vi "Save to ActiveX Excel - v2b.vi"(0 "Path":path caption="Excel Path", 1 "Excel._SheetName":string, 2 "ErrorIn":errorcluster, 3 "Ikol":i32, 4 "Table Mean Data":dbl[][](array[numeric])=[[0.03982848859388113, 0.8783843747615788, 1.7307777523460754, 2.548700999465932, 3.364561226825355], [0.09683070115205593, 0.9242182040131244, 1.7732014953841466, 2.5928838025482537, 3.4105195696955795], [0.13037125200274627, 0.9741591515983836, 1.8122639810788133, 2.646598611429008, 3.4407147325856373], [0.3228925001907382, 1.1797897306782663, 2.005814297703518, 2.8300938429846627, 3.6218649576562103], [0.3520146486610215, 1.202849774929428, 2.0447998779278245, 2.863716182192717, 3.6558284885938757], [1.3171953917753891, 2.1611230640115955, 2.9585827420462296, 3.7653595788509917, 4.528567025253687], [1.462092622262916, 2.2864551766231758, 3.104032959487296, 3.888673838406958, 4.6586440833142655], [1.5022079804684525, 2.335135728999771, 3.1296809338521387, 3.9336214236667435, 4.6988430609598], [1.5266187533379127, 2.364577096208133, 3.181790493629352, 3.9747548638132284, 4.713216449225604], [1.579623102159153, 2.4058289463645393, 3.208687266346226, 3.998727397573815, 4.759391470206768], [1.5989642175936543, 2.438834210727091, 3.2499842832074437, 4.027358205539025, 4.791335317006178], [1.6367565423056383, 2.4624704356450744, 3.273314106965741, 4.061460288395512, 4.821456626230265], [1.671589227130543, 2.5053598840314315, 3.307654840924691, 4.078201876859696, 4.83912291142138], [1.9548839551384747, 2.773676356145566, 3.5854721904325912, 4.353372701609829, 5.09703150988022], [1.9735957885099578, 2.8088496223392054, 3.6178268101014686, 4.38579995422294, 5.1040573739223385], [2.0215237659266037, 2.8251621271076495, 3.645978484779123, 4.413374227512019, 5.154262607766843], [2.063611200122071, 2.874846112764169, 3.6707408255130813, 4.4413080033569905, 5.182666971847107], [2.079061264972915, 2.9107945372701596, 3.7083878843366103, 4.474929121843292, 5.207357900358588], [2.3204461738002595, 3.1260236514839432, 3.9160466926070003, 4.67015243762875, 5.400686655985356], [2.4909175249866458, 3.2829407186999267, 4.078123140306708, 4.827607843137255, 5.545498435950253], [2.5371688410772846, 3.333136186770425, 4.0956087586785666, 4.86724528877699, 5.5768307011520575], [2.5549810025177377, 3.3498875410086164, 4.146593423361565, 4.901781948577098, 5.606005340657667], [2.593616845960172, 3.384173342488744, 4.175310292210271, 4.926442969405671, 5.625553368429085], [2.619952697032122, 3.4272117189288145, 4.190040131227593, 4.949809414816512, 5.647464713511864], [2.653675135423816, 3.450658121614398, 4.245682459754332, 4.983065537499049, 5.691289234760052], [2.856990615701531, 3.658316319523915, 4.410946211947819, 5.168084229800873, 5.859205615320062], [2.8970571450369995, 3.693769130998695, 4.459168383306632, 5.196810254062712, 5.892754711223012], [2.9354152742809165, 3.724582589456009, 4.481760280766007, 5.235593804837112, 5.9293153276874975], [4.518166475928902, 5.240471808957046, 5.927615472648206, 6.580137026016633, 7.176726939803161], [4.664593881132227, 5.399151598382549, 6.073597314412142, 6.700255436026549, 7.293027542534518], [4.6941597619592645, 5.413944914930952, 6.0971688410772895, 6.732541084916453, 7.310430151827263], [4.72799206530862, 5.443506523231869, 6.131480888075072, 6.7552147707331915, 7.341015335316998], [4.7442490272373625, 5.474857709620816, 6.148384832532239, 6.7895329213397355, 7.36304692149233], [4.777299458304725, 5.499158617532617, 6.170540321965362, 6.816587167162586, 7.378775310902568], [4.798946517128253, 5.526323338673995, 6.192271610589764, 6.82118928816662, 7.387563897154188], [4.901620202944993, 5.615843137254902, 6.292097352559698, 6.903707026779581, 7.473250629434656], [4.92828442816816, 5.6507722590981935, 6.304925917448693, 6.934254978255892, 7.480664072632936], [4.969151140611893, 5.675261158159765, 6.339691462577246, 6.9630627908751, 7.530664835584031], [5.006560158693834, 5.692798657206076, 6.368715953307389, 6.9916246280613334, 7.535613031204692], [5.044118715190357, 5.727861448081179, 6.395839169909206, 7.010927901121539, 7.563150072480349], [5.057027237354088, 5.78310582131685, 6.423008773937592, 7.0214792095826635, 7.583959105821311], [5.089166399633788, 5.78664469367514, 6.443226367589837, 7.063651483939874, 7.6117824063477455], [5.118777447165641, 5.826187533379106, 6.48167971313039, 7.071441519798577, 7.6265043106736785], [5.147915465018696, 5.842330357824063, 6.504778820477606, 7.0906581216144, 7.640489509422445], [5.195048142214084, 5.883804379339284, 6.519934691386284, 7.136523079270609, 7.677748378728906], [5.348665598535132, 6.047138780804155, 6.676741893644613, 7.253650110627901, 7.78973495078965], [5.394423743038073, 6.086649881742575, 6.72477546349278, 7.303063096055544, 7.841829861905848], [5.41259601739528, 6.1073417257953695, 6.748100404364077, 7.307313649195082, 7.860812085145335]]) -> (5 "error out":errorcluster, 6 "OK":bool)   [LabVIEW 2018]
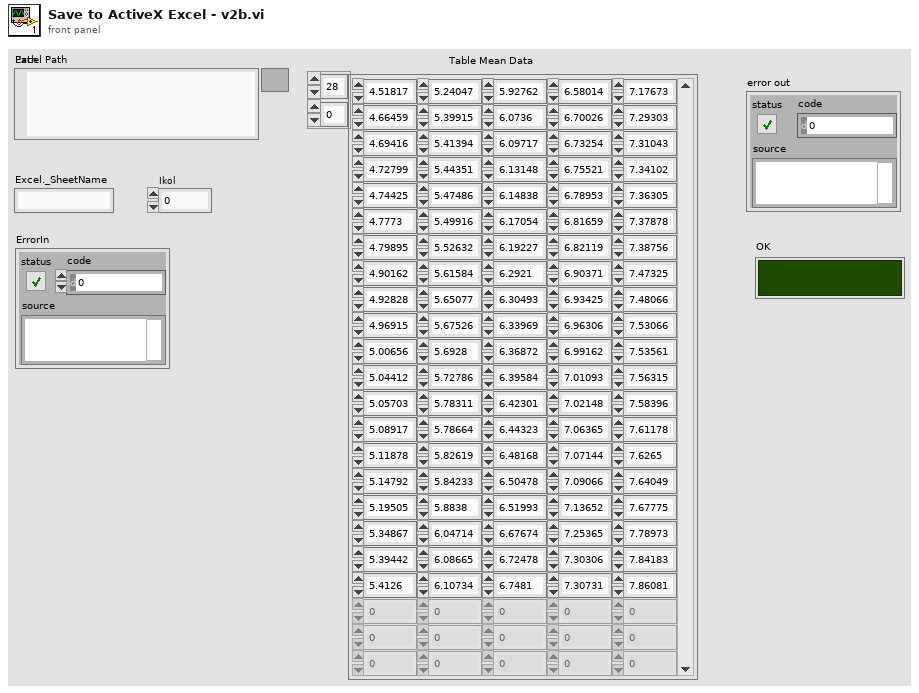
[diagram p1: front panel]
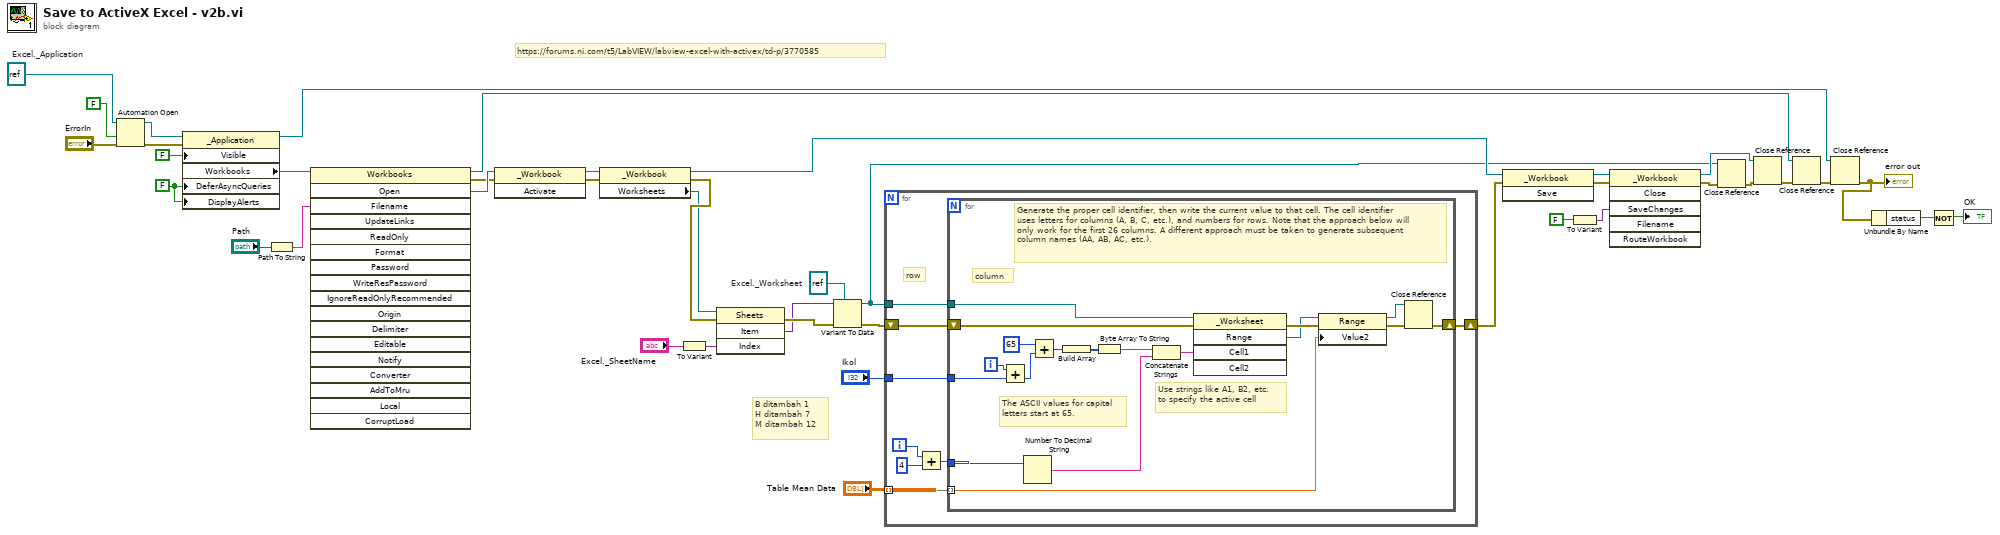
[diagram p0: block diagram]
diagram:
  w10 = refnum<k7> refnum  # Excel._Worksheet
  w41 = FALSE ("DeferAsyncQueries")
  w37 = refnum<k7> refnum  # Excel._Application
  # "B ditambah 1\nH ditambah 7\nM ditambah 12"
  # "https://forums.ni.com/t5/LabVIEW/labview-excel-with-activex/td-p/3770585"
  n1 = Automation Open(error in (no error)="ErrorIn", Automation Refnum=w37, 9:FALSE ("open new instance (false)")) -> (Automation Refnum=w39:refnum<k7>, error out=w38:errorcluster)  [unwired: 1 out]
  n2 = property class="_Application"(reference=w39, error in=w38, "Visible"=FALSE, "DeferAsyncQueries"=w41, "DisplayAlerts"=w41) -> (reference out=w17:refnum<k7>, "Workbooks"=w33:refnum<k7>)  [unwired: 1 out]
  n3 = Path To String(path="Path") -> (string=w30:string)
  n4 = invoke class="Workbooks" method="Open"(reference=w33, "Filename"=w30) -> (reference out=w19:refnum<k7>, error out=w34:errorcluster, "Open"=w35:refnum<k7>)  [unwired: 16 in, 15 out]
  n5 = invoke class="_Workbook" method="Activate"(reference=w35, error in=w34) -> (reference out=w29:refnum<k7>, error out=w28:errorcluster)  [unwired: 1 in, 1 out]
  n6 = property class="_Workbook"(reference=w29, error in=w28) -> (reference out=w27:refnum<k7>, error out=w4:errorcluster, "Worksheets"=w3:refnum<k7>)
  n7 = To Variant(anything="Excel._SheetName") -> (Variant=w6:variant)
  n8 = invoke class="Sheets" method="Item"(reference=w3, error in=w4, "Index"=w6) -> (error out=w5:errorcluster, "Item"=w2:variant)  [unwired: 1 in, 2 out]
  n9 = Variant To Data(error in=w5, type=w10, Variant=w2) -> (data=w8:refnum<k7>, error out=w12:errorcluster)
  n10 = for {
    shift-right: [w48] -> w9
    shift-left: w12 -> [w49]
    tunnel: w8 -> [w47]
    tunnel: "Table Mean Data" -> [w45] mode=indexing
    tunnel: "Ikol" -> [w42]
    i -> [w44]
    # "row"
    n11 = Add(x=w44, y=4) -> (x+y=w46:i32)
    n12 = for {
      shift-right: [w64] -> w48
      shift-left: w49 -> [w62]
      tunnel: w47 -> [w61]
      tunnel: w46 -> [w57]
      tunnel: w45 -> [w53] mode=indexing
      tunnel: w42 -> [w50]
      i -> [w51]
      # "column"
      # "Use strings like A1, B2, etc. to specify the active cell"
      # "The ASCII values for capital letters start at 65."
      # "Generate the proper cell identifier, then write the current value to that cell. The cell identifier uses letters for columns (A, B, C, etc.), and numbers for rows. Note that the approach below will only work for the first 26 columns. A different approach must be taken to generate subsequent column names (AA, AB, AC, etc.)."
      n13 = Add(x=w51, y=w50) -> (x+y=w52:i32)
      n14 = Number To Decimal String(number=w57) -> (decimal integer string=w55:string)  [unwired: 1 in]
      n15 = Add(x=65, y=w52) -> (x+y=w59:i32)
      n16 = Build Array(w59) -> (w58:i32[])
      n17 = Byte Array To String(unsigned byte array=w58) -> (string=w56:string)
      n18 = Concatenate Strings(w56, w55) -> (w54:string)
      n19 = invoke class="_Worksheet" method="Range"(reference=w61, error in=w62, "Cell1"=w54) -> (error out=w67:errorcluster, "Range"=w66:refnum<k7>)  [unwired: 2 in, 3 out]
      n20 = property class="Range"(reference=w66, error in=w67, "Value2"=w53) -> (reference out=w63:refnum<k7>, error out=w65:errorcluster)
      n21 = Close Reference(reference=w63, error in (no error)=w65) -> (error out=w64:errorcluster)
    }
  }
  n22 = invoke class="_Workbook" method="Save"(reference=w27, error in=w9) -> (reference out=w25:refnum<k7>, error out=w26:errorcluster)  [unwired: 1 in, 1 out]
  n23 = To Variant(anything=FALSE) -> (Variant=w23:variant)
  n24 = invoke class="_Workbook" method="Close"(reference=w25, error in=w26, "SaveChanges"=w23) -> (reference out=w21:refnum<k7>, error out=w15:errorcluster)  [unwired: 3 in, 4 out]
  n25 = Close Reference(reference=w8, error in (no error)=w15) -> (error out=w22:errorcluster)
  n26 = Close Reference(reference=w21, error in (no error)=w22) -> (error out=w20:errorcluster)
  n27 = Close Reference(reference=w19, error in (no error)=w20) -> (error out=w18:errorcluster)
  n28 = Close Reference(reference=w17, error in (no error)=w18) -> (error out=w16:errorcluster)
  "error out" <- w16
  n29 = Unbundle By Name(w16) -> ("status"=w14:bool)
  n30 = Not(x=w14) -> (.not. x?=→"OK":bool)
